vi "segment.vi"(8 "error in (no error)":errorcluster, 9 "ImageCollection in":refnum<class "ImageCollection.lvclass">[](array[class]), 10 "image file path":path, 11 "GenericSegmenter in":refnum<class "GenericSegmenter.lvclass">) -> (0 "error out":errorcluster, 1 "ImageCollection out":refnum<class "ImageCollection.lvclass">[](array[class]), 2 "segmented image path out":path, 3 "GenericSegmenter out":refnum<class "GenericSegmenter.lvclass">, 4 "centroids":T1[](array[typedef]))   [LabVIEW 2010, in "GenericSegmenter.lvclass"]
uses:
  GenericSegmenter.lvclass
  common/classes/ImageCollection/ImageCollection/ImageCollection.lvclass
  centroid_cluster.ctl
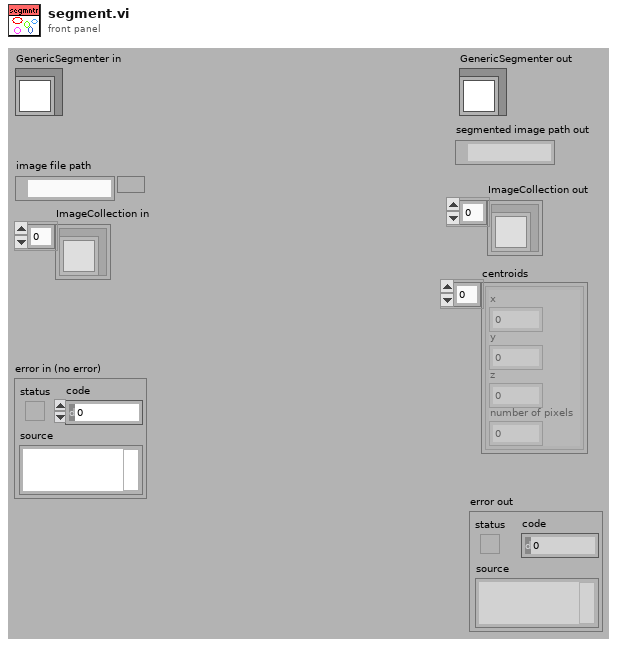
[diagram p1: front panel]
types:
  T1 = typedef "GenericSegmenter.lvclass/centroid_cluster.ctl" = cluster{"x":i32, "y":i32, "z":i32, "number of pixels":i32}
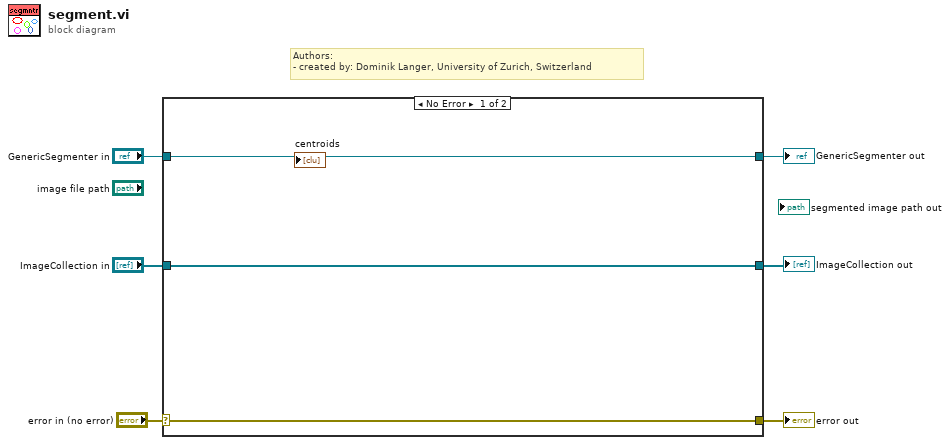
[diagram p0: block diagram]
diagram:
  # "Authors: \n- created by: Dominik Langer, University of Zurich, Switzerland"
  n1 = case shown="No Error" "error in (no error)" {
    selector: "error in (no error)" -> [w8 w12]
    tunnel: [w8 w12] -> w5
    tunnel: [w9 w11] -> w3
    tunnel: "GenericSegmenter in" -> [w9 w11]
    tunnel: "ImageCollection in" -> [w7 w10]
    tunnel: [w7 w10] -> w1
    frame No Error {
    }
    frame Error {
    }
  }
  "error out" <- w5
  "GenericSegmenter out" <- w3
  "ImageCollection out" <- w1
